vi "簇函数.vi"() -> ()   [LabVIEW 2010]
panel:
  out "温度数据":dbl
  out "状态":bool
  out "操作员":string
  out "插接的簇数组":cluster{i32, bool, string}[](array[cluster])=[{0, FALSE, "a"}, {1, TRUE, "b"}, {2, FALSE, "c"}]
  out "簇数组":cluster{i32[]}[](array[cluster])=[{[0, 1, 2]}, {[3, 4, 5]}, {[6, 7, 8]}]
  out "替换后的簇":cluster{"数值":i32, "字符":string, "逻辑":bool}
  out "字符":string
  out "数值":i32
  out "合成的簇":T1 {"?" format="%.2f"}
  out "替换后的簇":cluster{i32, string, bool}
  out "捆绑成的簇":cluster{i32, string, bool}
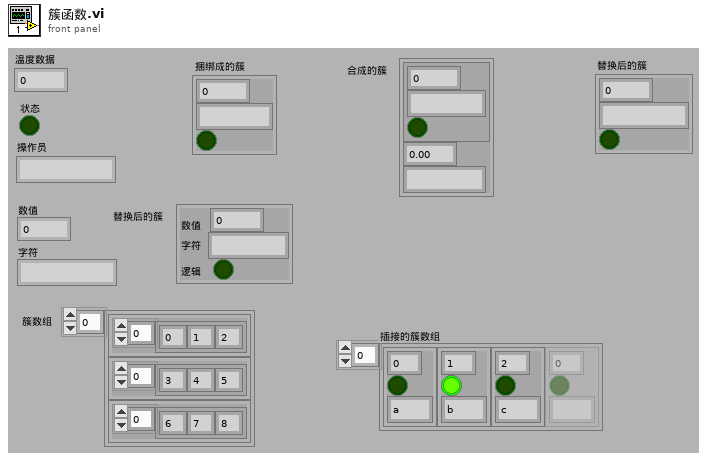
[diagram p1: front panel]
types:
  T1 = cluster{"攒成的簇":cluster{i32, string, bool}, dbl, "element":string}
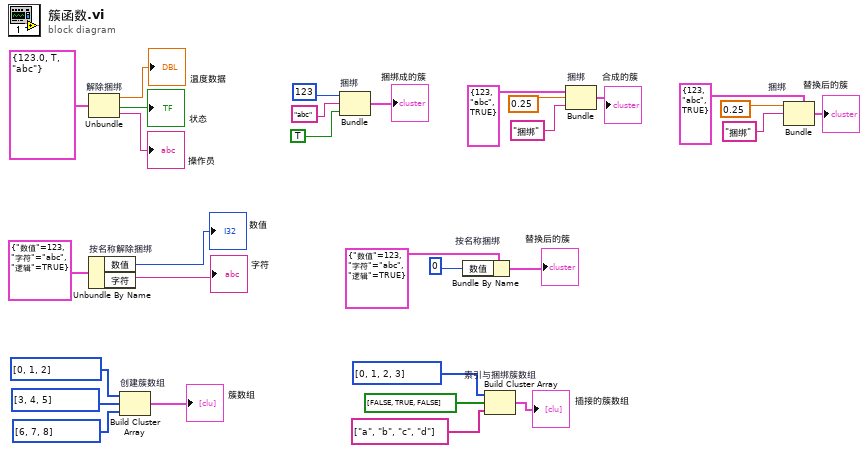
[diagram p0: block diagram]
diagram:
  n1 = Unbundle "解除捆绑"(cluster{"温度数据":dbl, "状态":bool, "操作员":string} {"温度数据"=123.0, "状态"=TRUE, "操作员"="abc"}) -> ("温度数据"=→"温度数据":dbl, "状态"=→"状态":bool, "操作员"=→"操作员":string)
  n2 = Unbundle By Name "按名称解除捆绑"(cluster{"数值":i32, "字符":string, "逻辑":bool} {"数值"=123, "字符"="abc", "逻辑"=TRUE} ("攒成的簇")) -> ("数值"=→"数值":i32, "字符"=→"字符":string)
  n3 = Build Cluster Array "创建簇数组"(i32[] [0, 1, 2], i32[] [3, 4, 5], i32[] [6, 7, 8]) -> (→"簇数组":cluster{i32[]}[])
  n4 = Bundle "捆绑"(123, "abc", TRUE) -> (→"捆绑成的簇":cluster{i32, string, bool})  [unwired: 1 in]
  n5 = Bundle By Name "按名称捆绑"(cluster=cluster{"数值":i32, "字符":string, "逻辑":bool} {"数值"=123, "字符"="abc", "逻辑"=TRUE} ("攒成的簇"), "数值"=0) -> (→"替换后的簇":cluster{"数值":i32, "字符":string, "逻辑":bool})
  n6 = Build Cluster Array "索引与捆绑簇数组"(i32[] [0, 1, 2, 3], bool[] [FALSE, TRUE, FALSE], string[] ["a", "b", "c", "d"]) -> (→"插接的簇数组":cluster{i32, bool, string}[])
  n7 = Bundle "捆绑"("攒成的簇"=cluster{i32, string, bool} {123, "abc", TRUE}, 0.25, "element"="捆绑") -> (→"合成的簇":T1)  [unwired: 1 in]
  n8 = Bundle "捆绑"(cluster=cluster{i32, string, bool} {123, "abc", TRUE} ("攒成的簇"), 0.25, "捆绑" ("element")) -> (→"替换后的簇":cluster{i32, string, bool})  [unwired: 1 in]
